vi "Get Config Path.vi"(8 "error in":errorcluster, 11 "Sequence Context In":refnum<k7>) -> (0 "error out":errorcluster, 2 "Configuration Path":path, 3 "Sequence Context out":refnum<k7>)   [LabVIEW 2023, in "Instrument Config.lvlib"]
uses:
  Instrument Config.lvlib
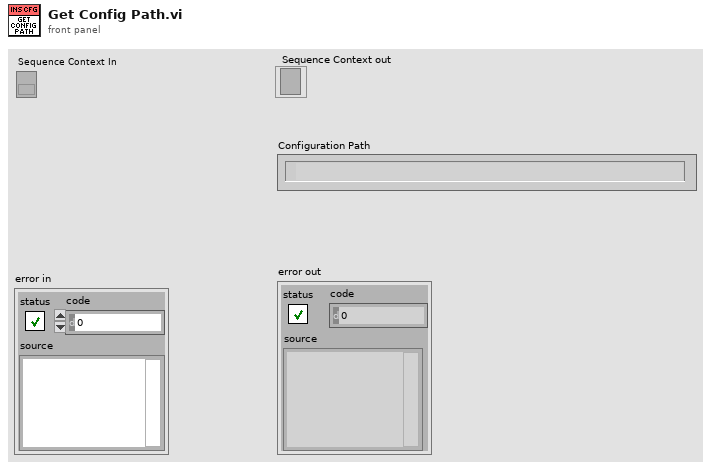
[diagram p1: front panel]
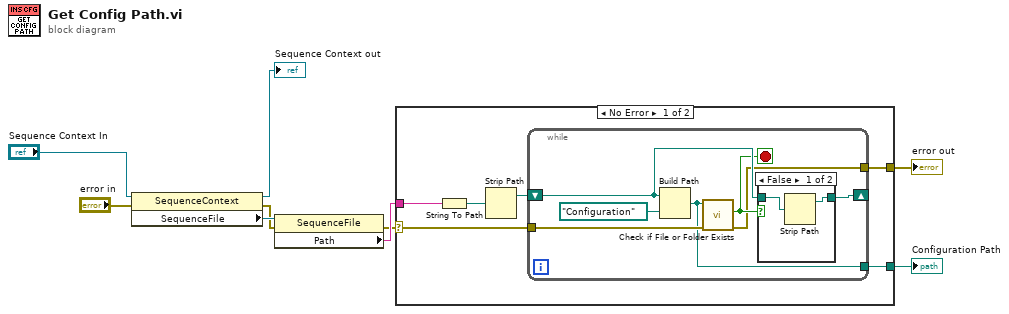
[diagram p0: block diagram]
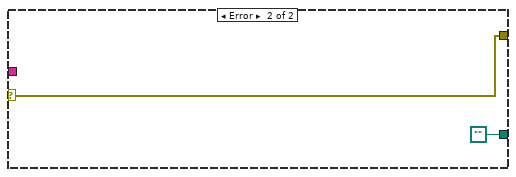
[diagram p3: hidden frame]
diagram:
  n1 = property class="SequenceContext"(reference="Sequence Context In", error in="error in") -> (reference out=→"Sequence Context out":refnum<k7>, error out=w6:errorcluster, "SequenceFile"=w7:refnum<k7>)
  n2 = property class="SequenceFile"(reference=w7, error in=w6) -> (error out=w2:errorcluster, "Path"=w5:string)  [unwired: 1 out]
  n3 = case shown="No Error" w2 {
    selector: w2 -> [w11 w27]
    tunnel: w5 -> [w15 _]
    tunnel: [w14 path ""] -> w3
    tunnel: [w10 w27] -> w1
    frame No Error {
      n4 = String To Path(string=w15) -> (path=w12:path)
      n5 = Strip Path(path=w12) -> (stripped path=w13:path)  [unwired: 1 out]
      n6 = while {
        shift-right: [w21] -> _
        shift-left: w13 -> [w20]
        tunnel: [w16] -> w14
        tunnel: w11 -> [w18]
        tunnel: [w17] -> w10
        stop <- w19 stop-if-true
        n7 = Build Path(base path=w20, name or relative path=path "Configuration") -> (appended path=w16:path)
        n8 = call <vilib>:"Check if File or Folder Exists.vi"("error in (no error)"=w18, "path"=w16) -> ("error out"=w17:errorcluster, "file or folder exists?"=w19:bool)  [unwired: 7 in, 1 out]
        n9 = case shown="False" w19 {
          tunnel: w20 -> [w24 w25]
          tunnel: [w23 w25] -> w21
          frame False {
            n10 = Strip Path(path=w24) -> (stripped path=w23:path)  [unwired: 1 out]
          }
          frame True {
          }
        }
      }
    }
    frame Error {
    }
  }
  "error out" <- w1
  "Configuration Path" <- w3
